vi "ExtendedRegisterWriteLong.vi"(7 "Extended Read/Write Long":T1 {"Data" format="%.0x"; "Register" format="%.0x"; "Slave Address" max=15 format="%.0x"}, 8 "error in (no error)":errorcluster, 9 "Number of Samples In":i32, 10 "Data Array":u8[][](array[numeric]), 11 "RFFE_Data":T2 {"Toggle (high to low)" items=["0", "1", "Z", "L", "H", "X", "T", "V"]; "X Array" items=["0", "1", "Z", "L", "H", "X", "T", "V"]; "Z Array" items=["0", "1", "Z", "L", "H", "X", "T", "V"]; "L Array" items=["0", "1", "Z", "L", "H", "X", "T", "V"]; "H Array" items=["0", "1", "Z", "L", "H", "X", "T", "V"]; "One Array" items=["0", "1", "Z", "L", "H", "X", "T", "V"]; "Zero Array" items=["0", "1", "Z", "L", "H", "X", "T", "V"]}) -> (0 "error out":errorcluster, 1 "Number of Samples Out out":i32, 2 "Data Array Out":u8[][](array[numeric]), 3 "Configuratation Out":T2 {"Toggle (high to low)" items=["0", "1", "Z", "L", "H", "X", "T", "V"]; "X Array" items=["0", "1", "Z", "L", "H", "X", "T", "V"]; "Z Array" items=["0", "1", "Z", "L", "H", "X", "T", "V"]; "L Array" items=["0", "1", "Z", "L", "H", "X", "T", "V"]; "H Array" items=["0", "1", "Z", "L", "H", "X", "T", "V"]; "One Array" items=["0", "1", "Z", "L", "H", "X", "T", "V"]; "Zero Array" items=["0", "1", "Z", "L", "H", "X", "T", "V"]})   [LabVIEW 2011]
doc: "Builds MIPI RFFE Extended Register Write Long with the specified data."
uses:
  Ctrls/RFFE_Data.ctl
  Ctrls/ClockDataChannels.ctl
  Ctrls/ExtendedRegReadWriteLong.ctl
  Ctrls/Commands.ctl
  Ctrls/Read_Write_Data.ctl
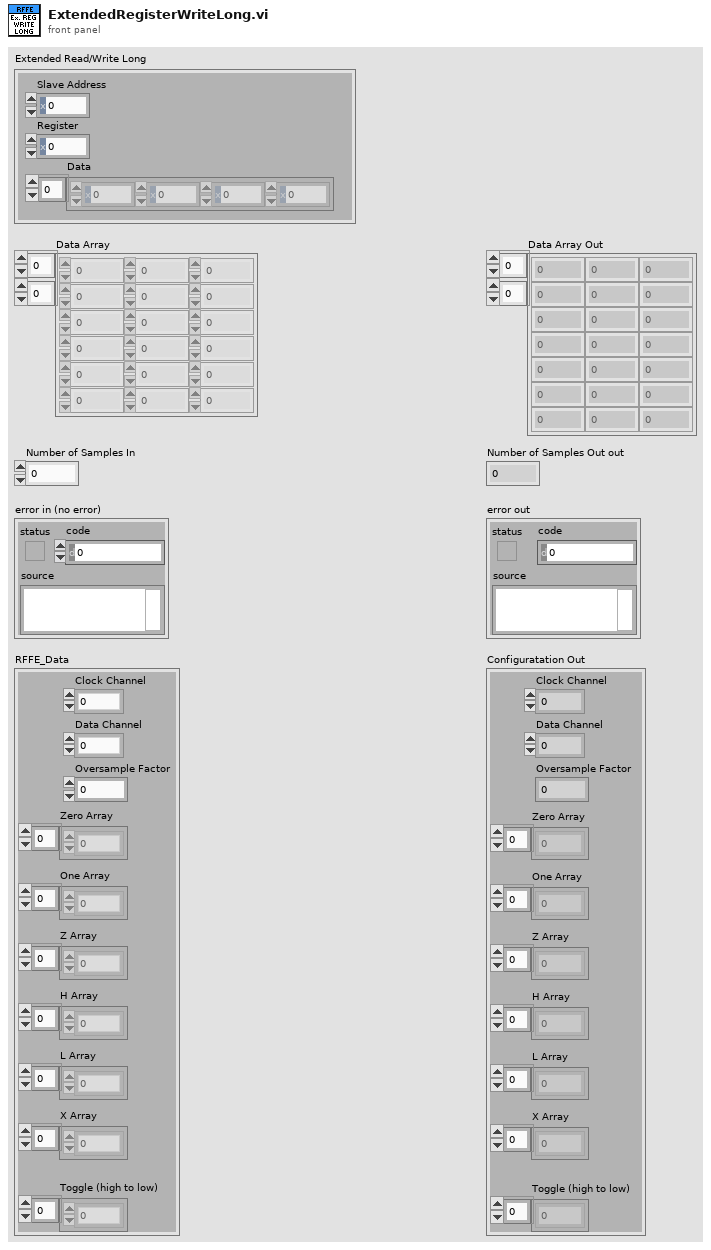
[diagram p1: front panel]
types:
  T1 = typedef "ExtendedRegReadWriteLong.ctl" = cluster{"Slave Address":u8, "Register":u16, "Data":u8[]}
  T2 = typedef "RFFE_Data.ctl" = cluster{"Clock Channel":T3, "Data Channel":T3, "Oversample Factor":u8, "Zero Array":u8[], "One Array":u8[], "Z Array ":u8[], "H Array":u8[], "L Array":u8[], "X Array":u8[], "Toggle (high to low)":u8[]}
  T3 = typedef "ClockDataChannels.ctl" = enum16{"0", "1"}
  T4 = typedef "Read_Write_Data.ctl" = cluster{"Data":u8, "Read/Write":enum16{"Read", "Write"}}
  T5 = typedef "Commands.ctl" = cluster{"Command":enum16{"Extended Register Write", "Extended Register Read", "Extended Register Write Long", "Extended Register Read Long", "Register Write", "Register Read", "Register 0 Write"}, "Data/Address/ByteCount":u8}
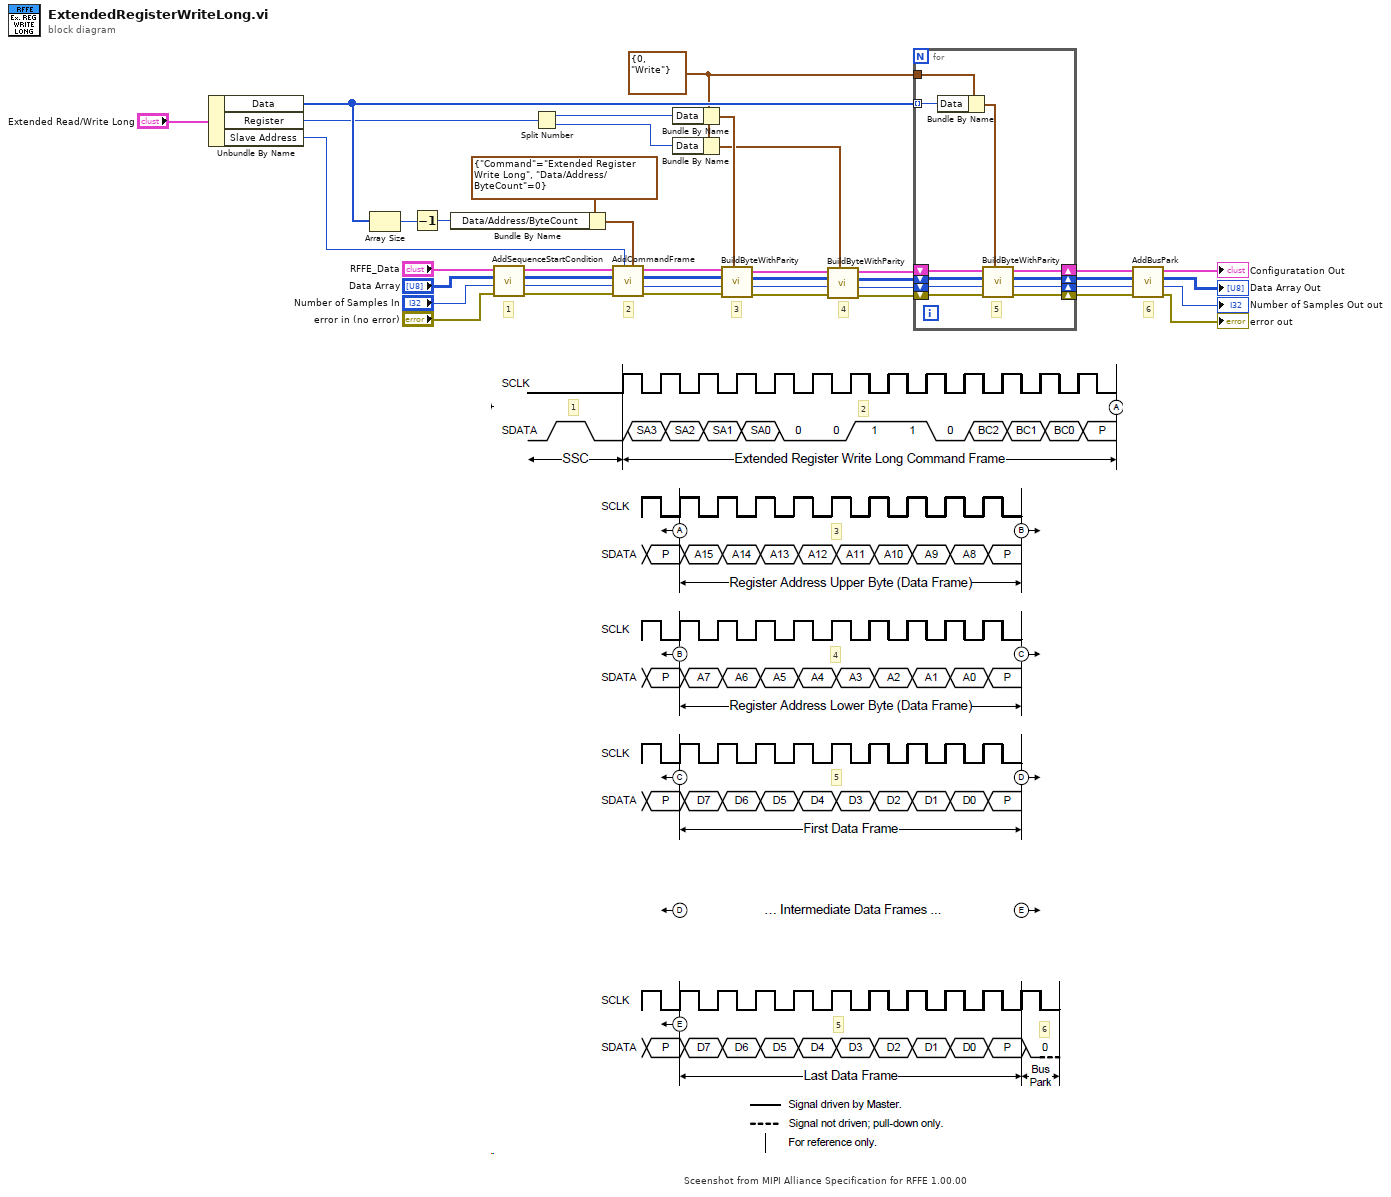
[diagram p0: block diagram]
diagram:
  w16 = T4 {"Data"=0, "Read/Write"=enum."Write"} ("Read/Write Data")
  # "Sceenshot from MIPI Alliance Specification for RFFE 1.00.00"
  # "5"
  # "6"
  # "5"
  # "4"
  # "3"
  # "2"
  # "1"
  # "6"
  # "4"
  # "3"
  # "2"
  # "1"
  n1 = Unbundle By Name("Extended Read/Write Long") -> ("Data"=w19:u8[], "Register"=w18:u16, "Slave Address"=w1:u8)
  n2 = Array Size(array=w19) -> (size(s)=w20:i32)
  n3 = Decrement(x=w20) -> (x-1=w4:i32)
  n4 = Bundle By Name(cluster=T5 {"Command"=enum."Extended Register Write Long", "Data/Address/ByteCount"=0} ("Command"), "Data/Address/ByteCount"=w4) -> (w2:T5)
  n5 = call "AddSequenceStartCondition.vi"("error in (no error)"="error in (no error)", "Number of Samples In"="Number of Samples In", "Data Array In"="Data Array", "RFFE_Data In"="RFFE_Data") -> ("error out"=w32:errorcluster, "Number of Samples Out"=w39:i32, "Data Array Out"=w33:u8[][], "RFFE_Data Out"=w34:T2)  [unwired: 4 in]
  n6 = Split Number(x=w18) -> (hi(x)=w17:u8, lo(x)=w15:u8)
  n7 = call "AddCommandFrame.vi"("Command"=w2, "Slave Address"=w1, "error in (no error)"=w32, "Number of Samples In"=w39, "Data Array In"=w33, "RFFE_Data"=w34) -> ("error out"=w35:errorcluster, "Number of Samples Out"=w37:i32, "Data Array Out"=w38:u8[][], "Configuratation Out"=w36:T2)  [unwired: 2 in]
  n8 = Bundle By Name(cluster=w16, "Data"=w17) -> (w6:T4)
  n9 = Bundle By Name(cluster=w16, "Data"=w15) -> (w5:T4)
  n10 = call "BuildByteWithParity.vi"("Read/Write Data"=w6, "error in"=w35, "Number of Samples In"=w37, "Data Array In"=w38, "RFFE_Data In"=w36) -> ("error out"=w14:errorcluster, "Number of Samples Out"=w12:i32, "Data Array Out"=w10:u8[][], "RFFE_Data Out"=w7:T2)  [unwired: 2 in, 1 out]
  n11 = call "BuildByteWithParity.vi"("Read/Write Data"=w5, "error in"=w14, "Number of Samples In"=w12, "Data Array In"=w10, "RFFE_Data In"=w7) -> ("error out"=w13:errorcluster, "Number of Samples Out"=w11:i32, "Data Array Out"=w9:u8[][], "RFFE_Data Out"=w8:T2)  [unwired: 2 in, 1 out]
  n12 = for {
    shift-right: [w51] -> w24
    shift-left: w13 -> [w52]
    shift-right: [w48] -> w21
    shift-left: w11 -> [w50]
    shift-right: [w47] -> w22
    shift-left: w9 -> [w49]
    shift-right: [w46] -> w23
    shift-left: w8 -> [w45]
    tunnel: w19 -> [w44] mode=indexing
    tunnel: w16 -> [w42]
    # "5"
    n13 = Bundle By Name(cluster=w42, "Data"=w44) -> (w43:T4)
    n14 = call "BuildByteWithParity.vi"("Read/Write Data"=w43, "error in"=w52, "Number of Samples In"=w50, "Data Array In"=w49, "RFFE_Data In"=w45) -> ("error out"=w51:errorcluster, "Number of Samples Out"=w48:i32, "Data Array Out"=w47:u8[][], "RFFE_Data Out"=w46:T2)  [unwired: 2 in, 1 out]
  }
  n15 = call "AddBusPark.vi"("error in (no error)"=w24, "Number of Samples In"=w21, "Data Array In"=w22, "RFFE_Data In"=w23) -> ("error out"=→"error out":errorcluster, "Number of Samples Out"=→"Number of Samples Out out":i32, "Data Array Out"=→"Data Array Out":u8[][], "RFFE_Data Out"=→"Configuratation Out":T2)  [unwired: 4 in]
